vi "InitConfig.vi"() -> ()   [LabVIEW 2014]
uses:
  QMH Fundamentals - Message Cluster.ctl
panel:
  in  "请选择使用的参数":u16(ring) items=["第一条", "第二条", "第三条", "第四条", "第五条"]
  out "保存的参数":string[][](table)
  in  "调用已有参数确定":bool
  in  "调用已有参数返回":bool
  in  "手动确定":bool
  in  "手动示波器试验频率设置(s/条)":dbl=10.0 min=10.0
  in  "示波器试验频率设置(s/条)":dbl=10000.0 min=10000.0
  out "创建的文件路径":string
  in  "请输入需要创建的文件夹名称":string
  in  "路径确定":bool
  in  "自定义试验时间设置(小时)":dbl=0.003 min=0.003
  in  "自定义确定":bool
  in  "自定义返回":bool
  in  "高温老练试验时间设置(小时)":dbl=0.003 min=0.003
  in  "高温老练返回":bool
  in  "高温老练确定":bool
  in  "温循返回":bool
  in  "温循确定":bool
  in  "温循试验时间设置(小时)":dbl=0.003 min=0.003
  in  "单次":bool
  in  "调用已有参数":bool
  in  "手动返回":bool
  in  "返回":bool
  in  "自定义":bool
  in  "高温老练":bool
  in  "温循":bool
  in  "退出":bool
  in  "手动测试":bool
  in  "自动测试":bool
  # "低压元器件应用验证测试系统"
  # "请确定输出文件路径(EXCEL)"
  # "请选择测试类型"
  # "基路径: C:\\output_xls\\"
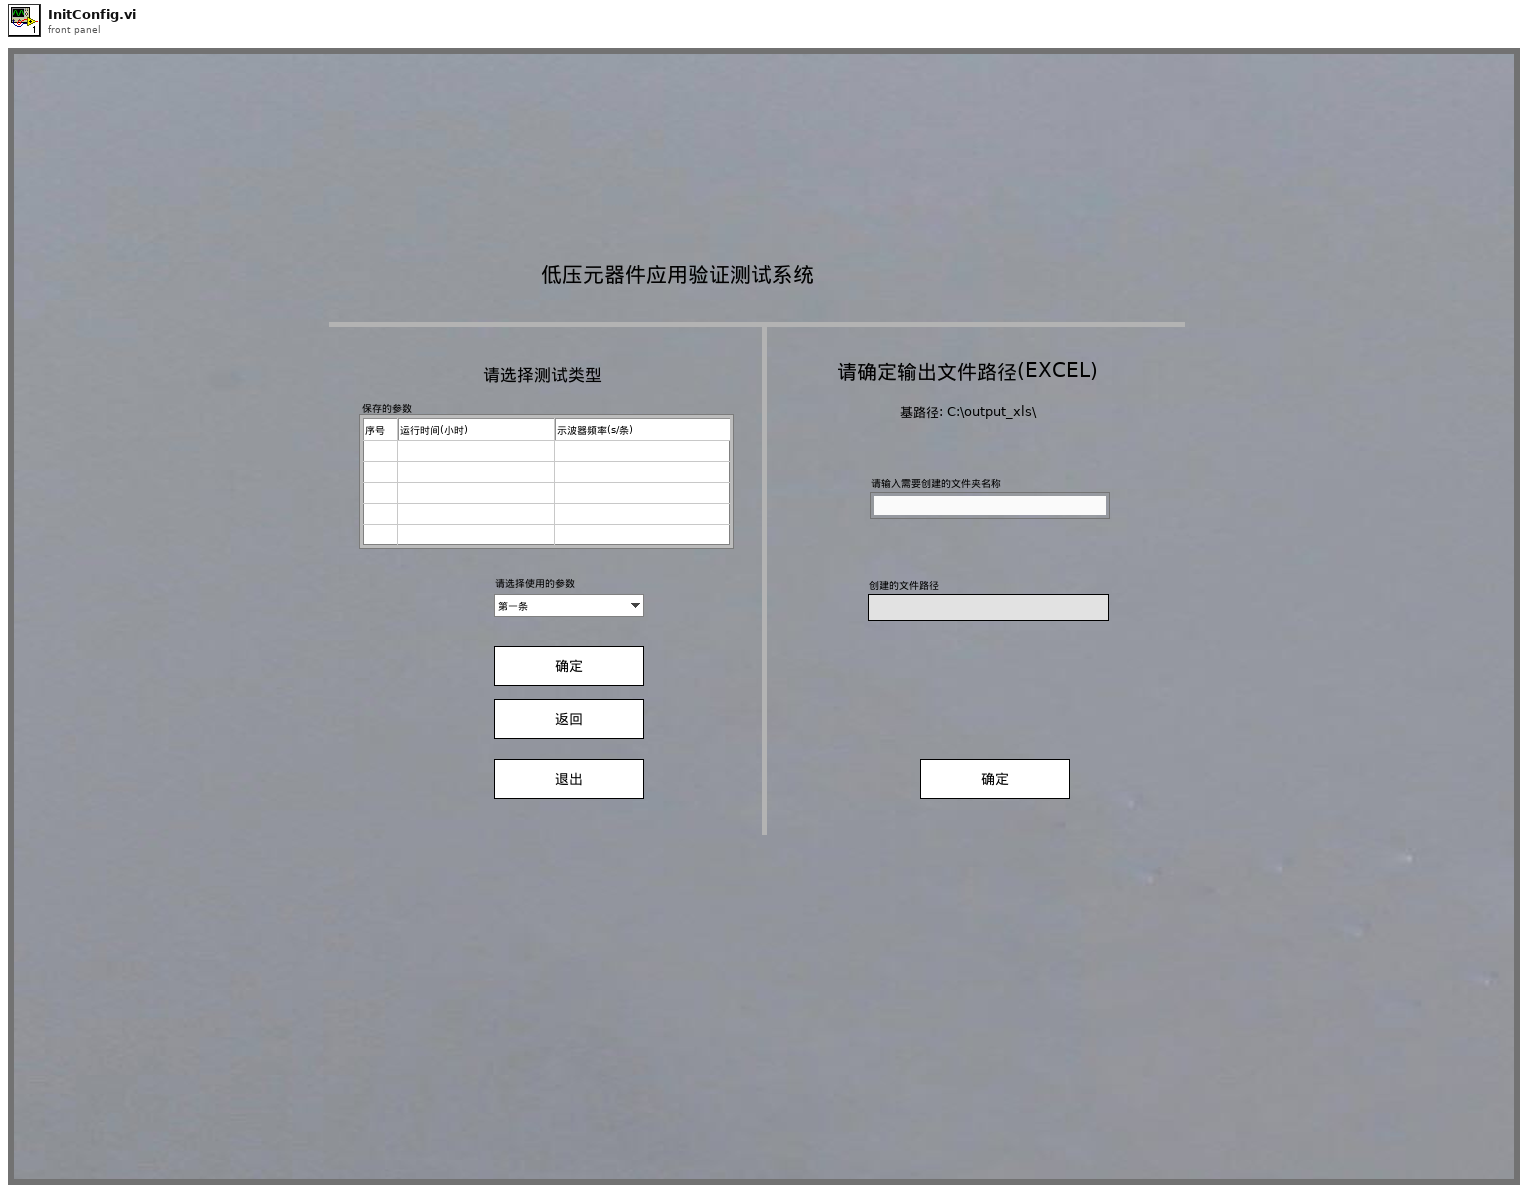
[diagram p1: front panel]
types:
  T1 = typedef "QMH Fundamentals - Message Cluster.ctl" = cluster{"消息":string, "消息数据":variant}
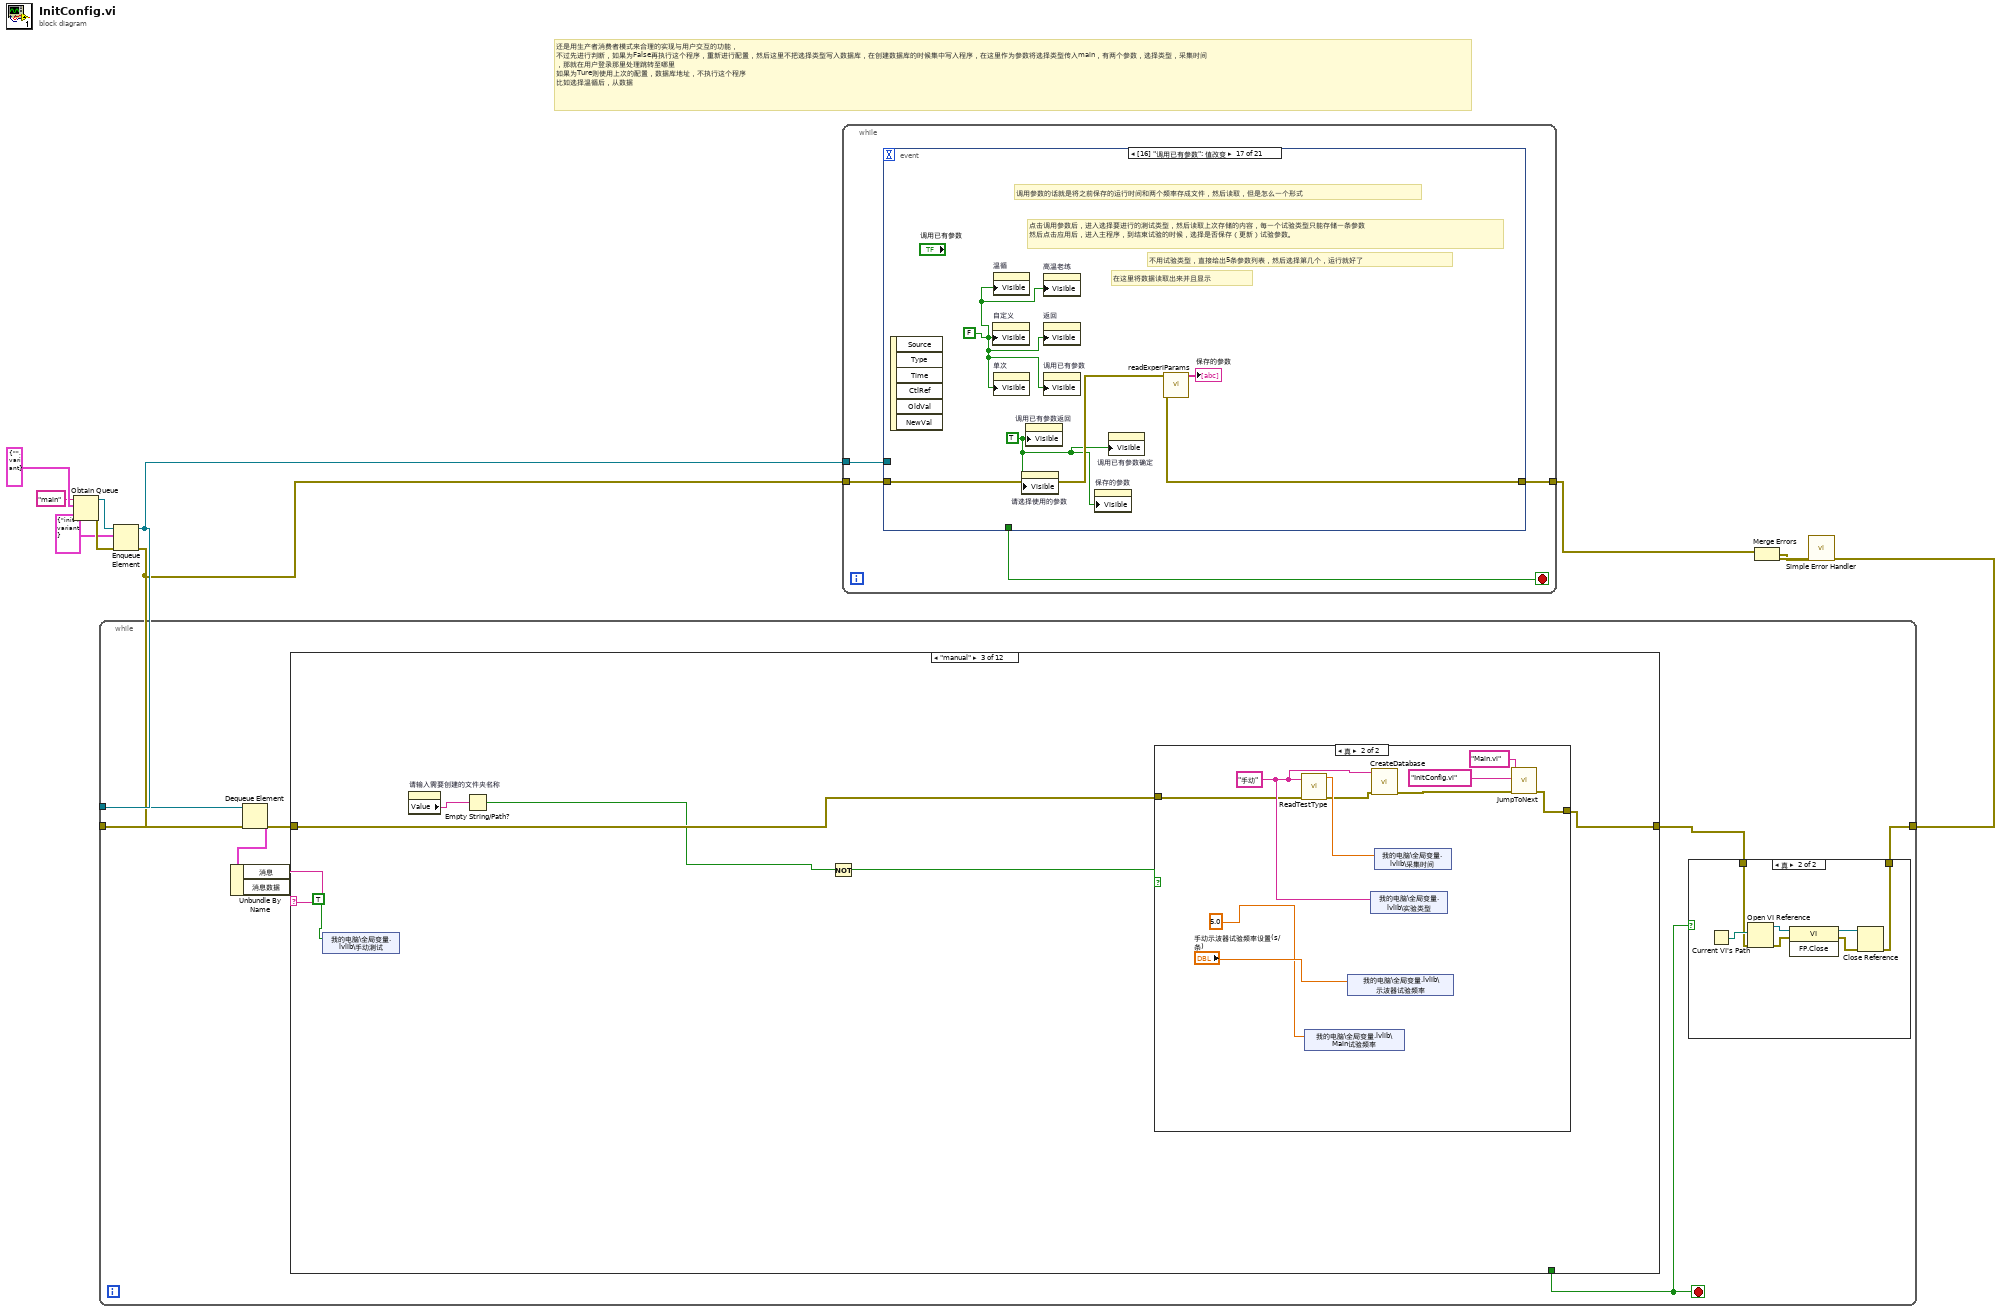
[diagram p0: block diagram]
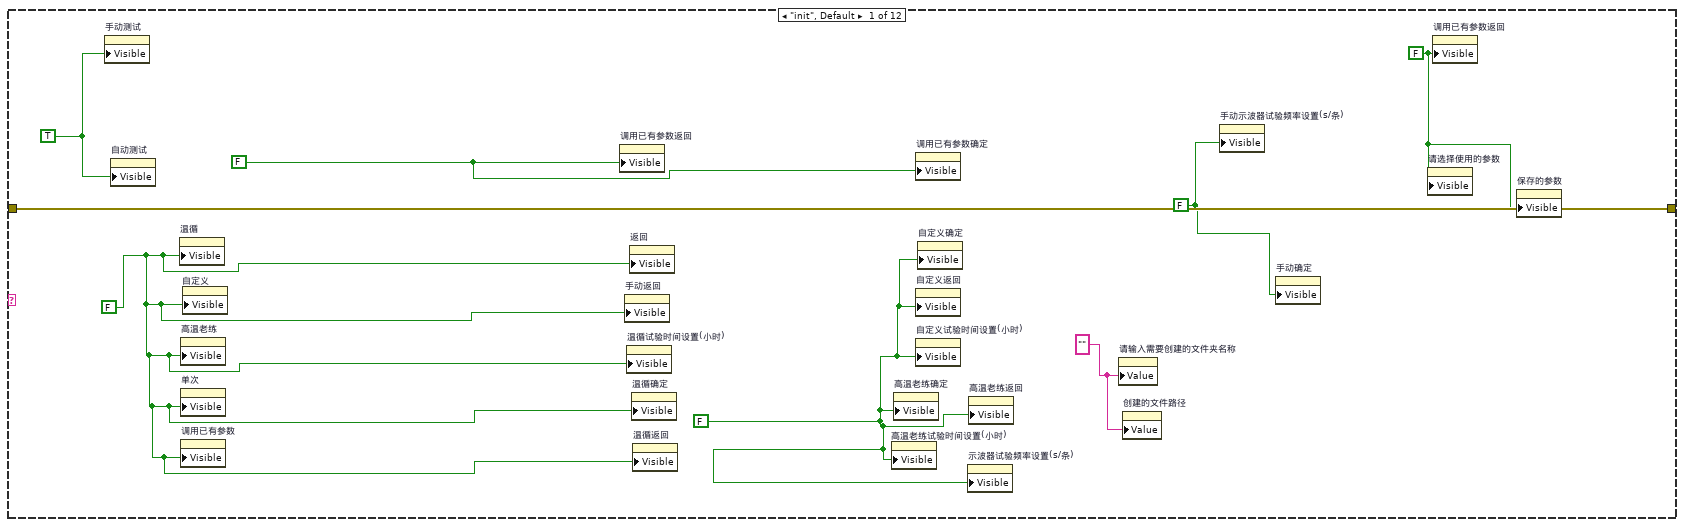
[diagram p3: hidden frame]
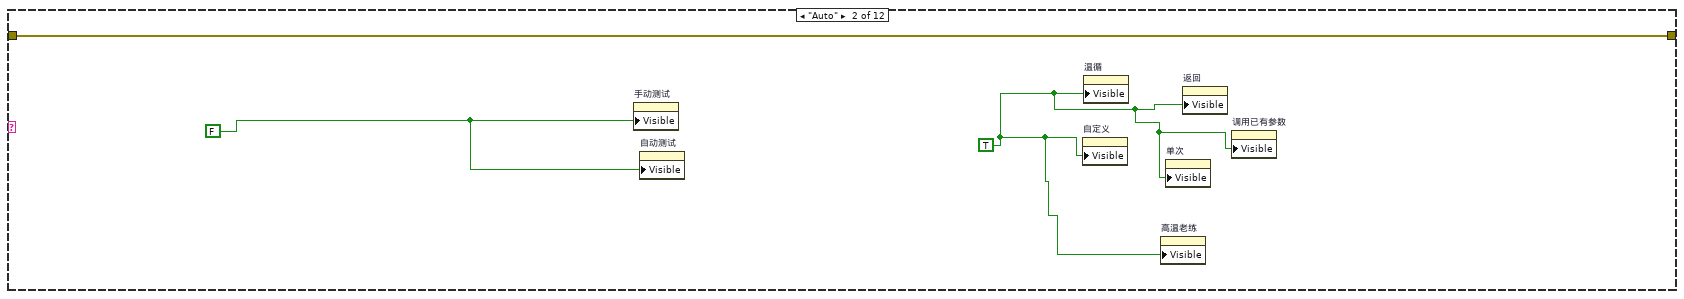
[diagram p4: hidden frame]
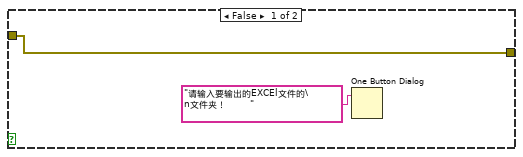
[diagram p5: hidden frame]
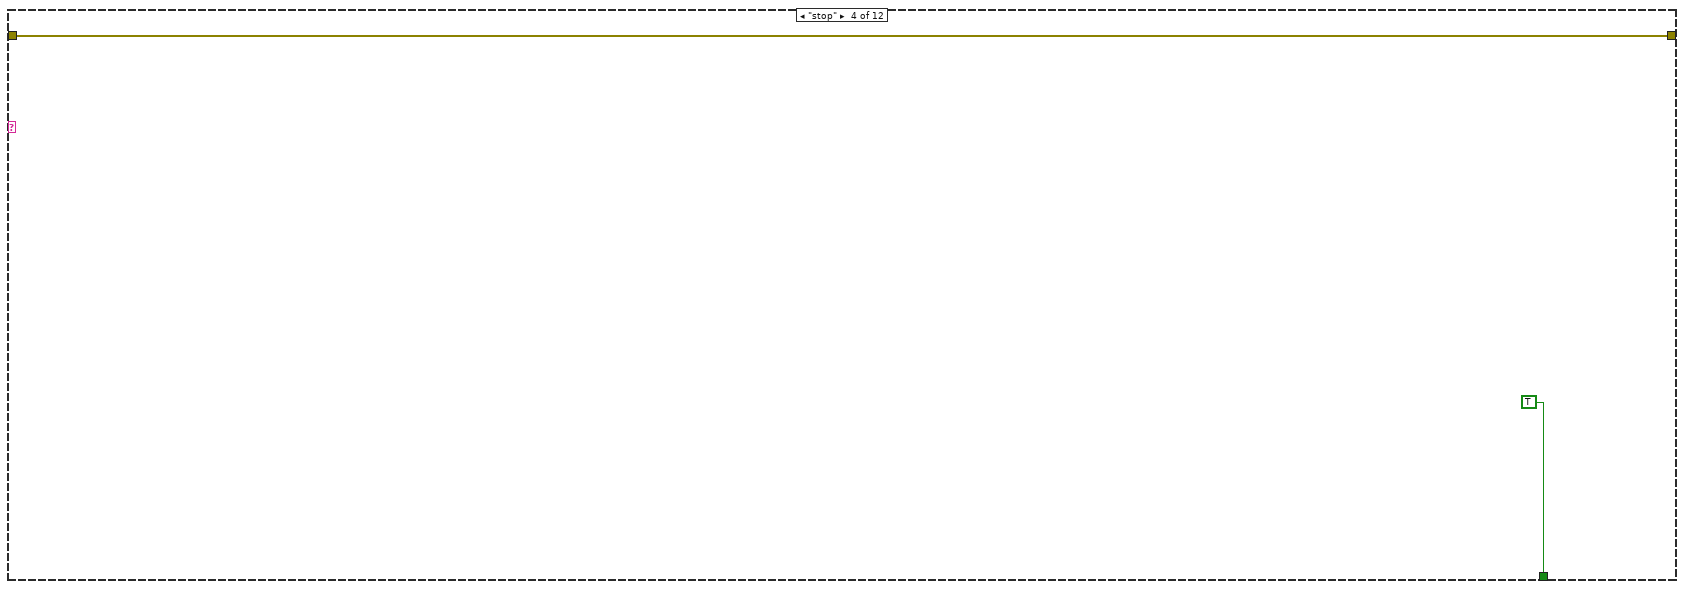
[diagram p6: hidden frame]
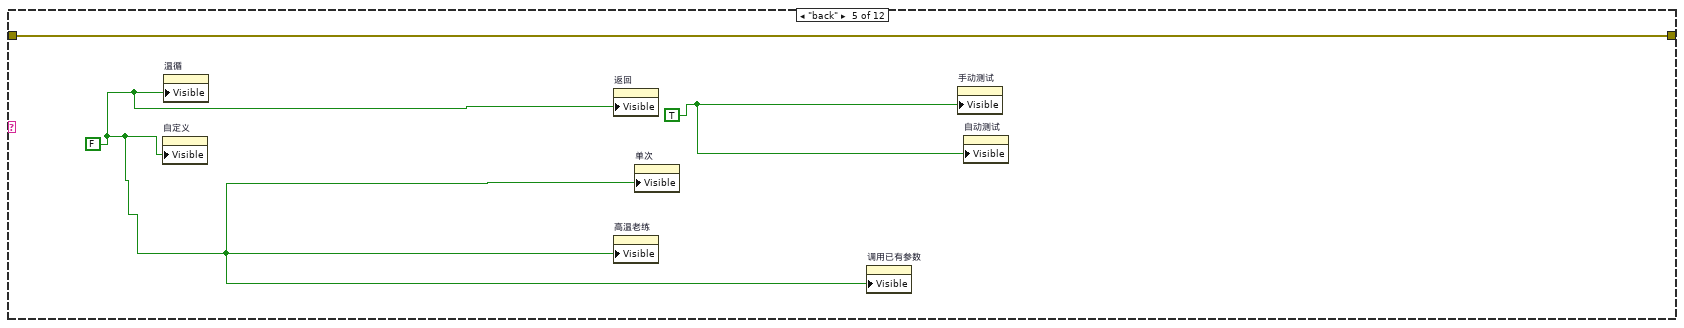
[diagram p7: hidden frame]
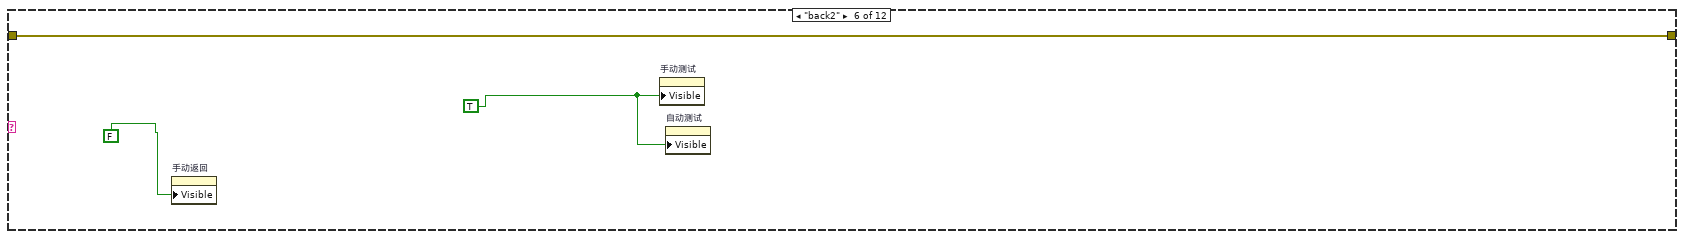
[diagram p8: hidden frame]
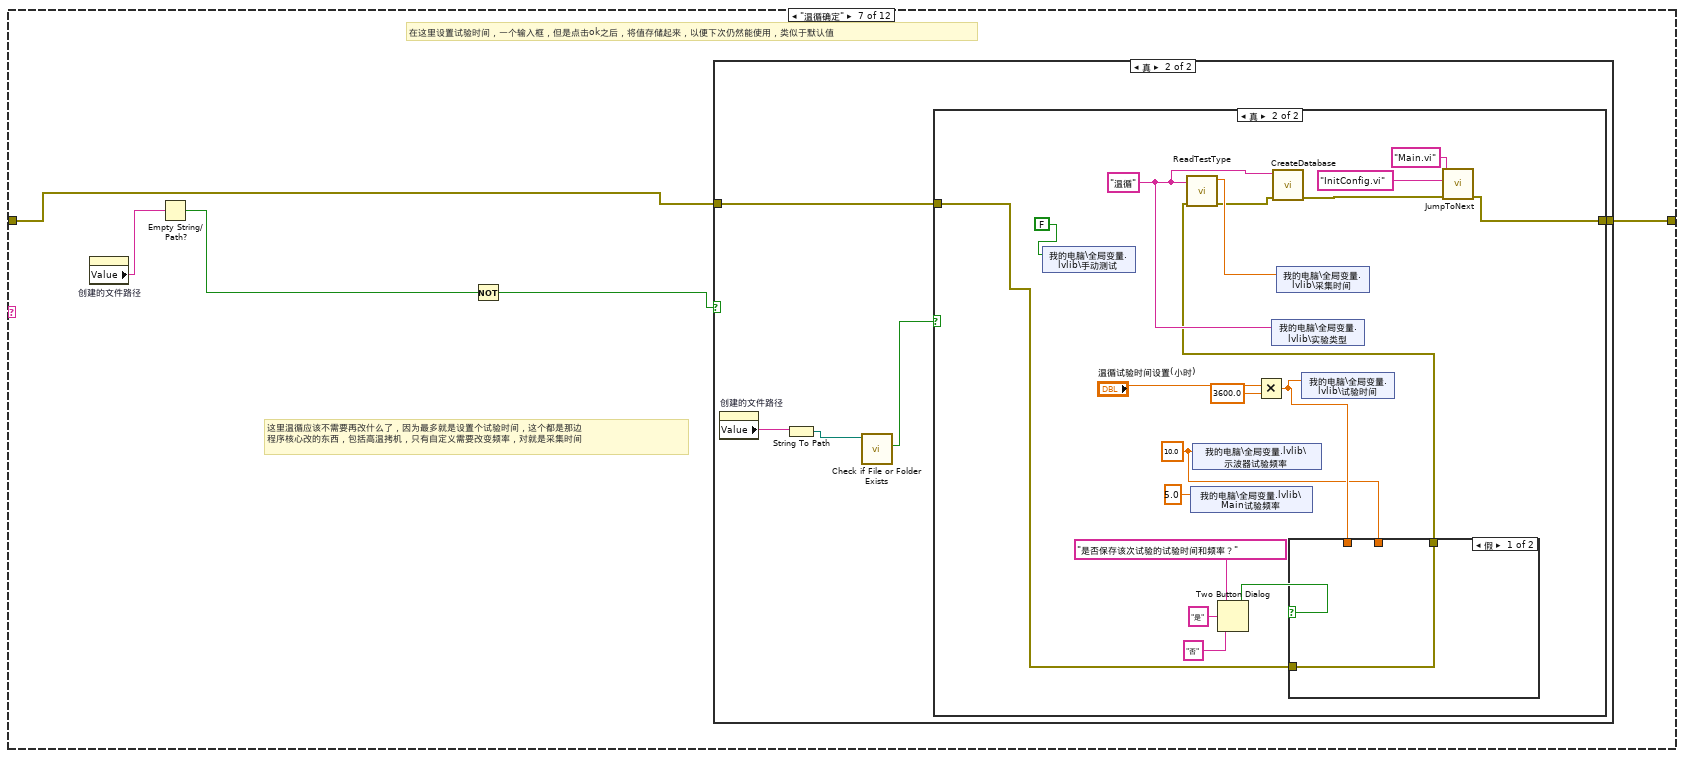
[diagram p9: hidden frame]
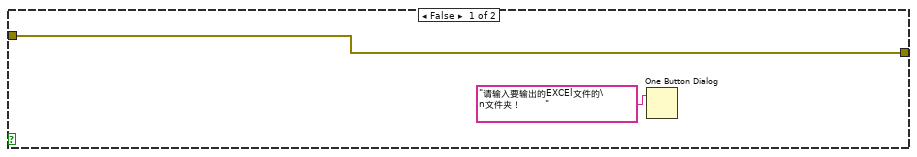
[diagram p10: hidden frame]
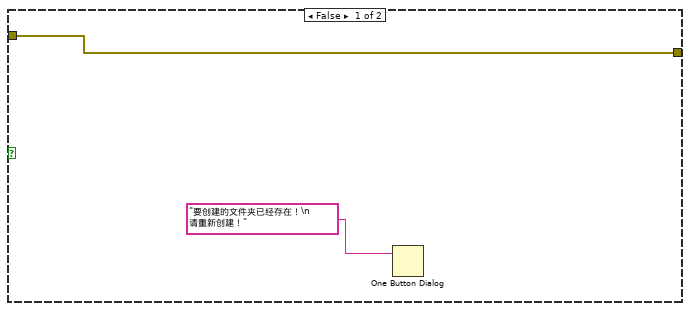
[diagram p11: hidden frame]
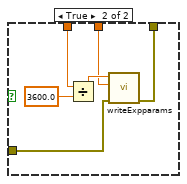
[diagram p12: hidden frame]
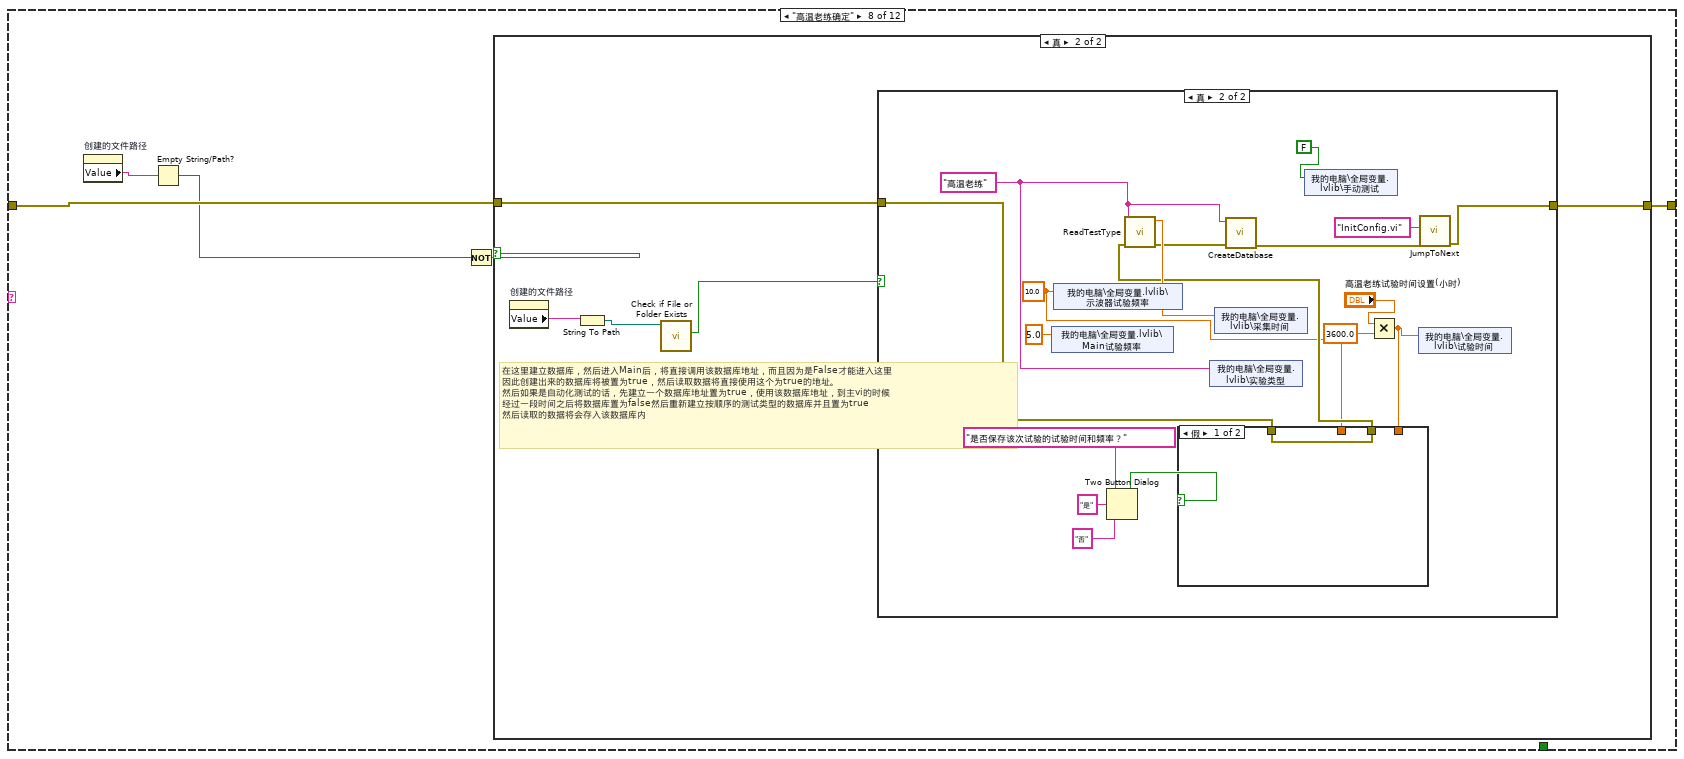
[diagram p13: hidden frame]
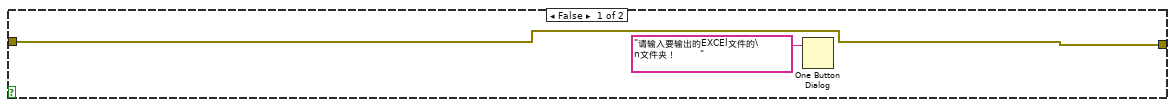
[diagram p14: hidden frame]
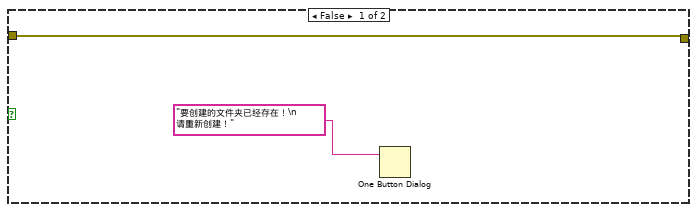
[diagram p15: hidden frame]
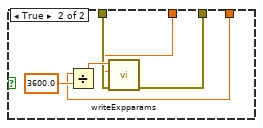
[diagram p16: hidden frame]
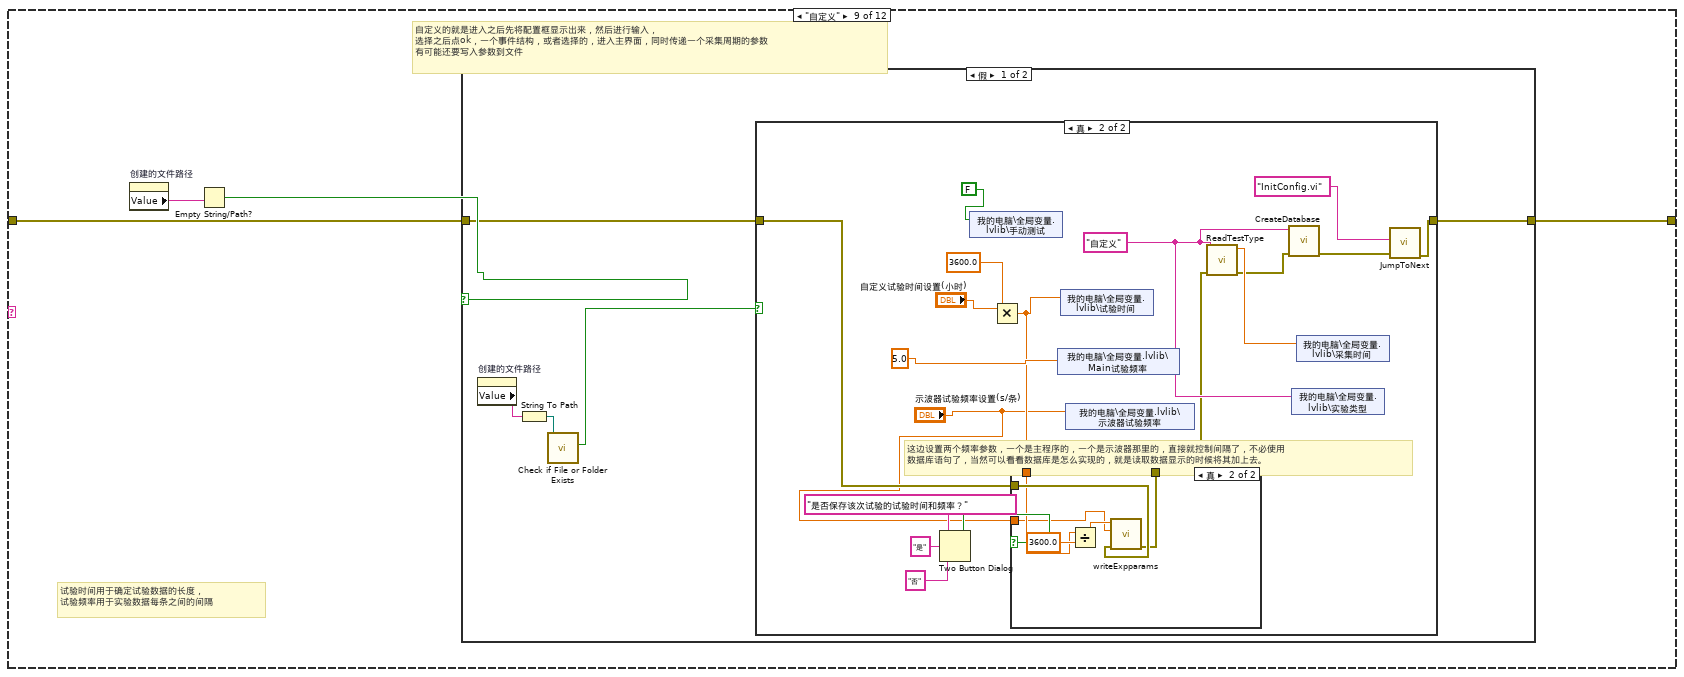
[diagram p17: hidden frame]
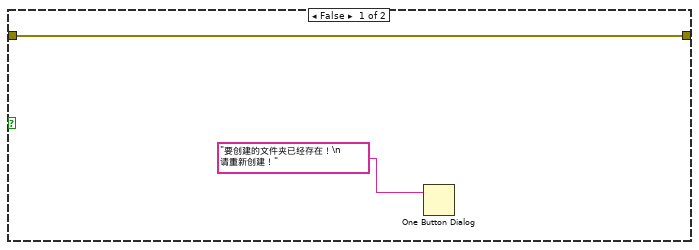
[diagram p18: hidden frame]
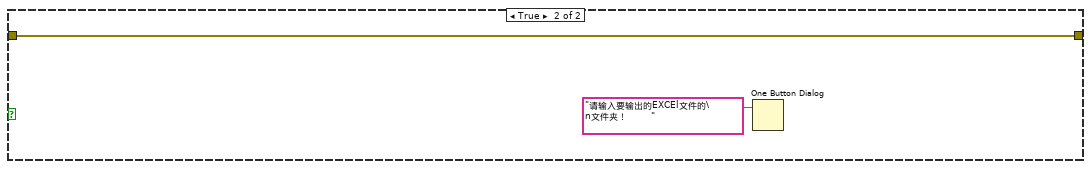
[diagram p20: hidden frame]
diagram:
  # "还是用生产者消费者模式来合理的实现与用户交互的功能，\n不过先进行判断，如果为False再执行这个程序，重新进行配置，然后这里不把选择类型写入数据库，在创建数据库的时候集中写入程序，在这里作为参数将选择类型传入main，有两个参数，选择类型，采集时间\n，那就在用户登录那里处理跳转至哪里\n如果为Ture则使用上次的配置，数据库地址，不执行这个程序\n比如选择温循后，从数据"
  n1 = Obtain Queue(name (unnamed)="main" ("名称（未命名）"), element data type=T1 {"消息"="", "消息数据"=variant} ("消息簇")) -> (queue out=w8:refnum<queue>, error out=w7:errorcluster)  [unwired: 3 in, 1 out]
  n2 = Enqueue Element(queue=w8, element=T1 {"消息"="init", "消息数据"=variant} ("元素"), error in (no error)=w7) -> (queue out=w5:refnum<queue>, error out=w4:errorcluster)  [unwired: 1 in, 1 out]
  n3 = while {
    tunnel: w5 -> [w18]
    tunnel: w4 -> [w17]
    tunnel: [w11] -> w2
    stop <- w13 stop-if-true
    n4 = Dequeue Element(queue=w18, error in (no error)=w17) -> (element=w16:T1, error out=w14:errorcluster)  [unwired: 1 in, 2 out]
    n5 = Unbundle By Name(w16) -> ("消息"=w15:string)  [unwired: 1 out]
    n6 = case shown="\"manual\"" w15 {
      tunnel: w14 -> [w34 w37 w40 w57 w59 w61 w68 w107 w146 w184 w218 w263]
      tunnel: [w34 w37 w39 w57 w59 w61 w67 w106 w145 w183 w219 w268] -> w12
      tunnel: [_ _ _ TRUE _ _ _ _ _ _ _ _] -> w13
      frame "init", Default {
        w28 = FALSE ("可见")
        w27 = FALSE ("可见")
        w29 = FALSE
        w31 = ""
        w30 = FALSE
        w33 = TRUE
        w32 = FALSE
        n7 = property on="手动测试" class="Bool"("Visible"=w33) -> ()  [unwired: 2 in, 2 out]
        n8 = property on="自动测试" class="Bool"("Visible"=w33) -> ()  [unwired: 2 in, 2 out]
        n9 = property on="温循" class="Bool"("Visible"=w32) -> ()  [unwired: 2 in, 2 out]
        n10 = property on="高温老练" class="Bool"("Visible"=w32) -> ()  [unwired: 2 in, 2 out]
        n11 = property on="单次" class="Bool"("Visible"=w32) -> ()  [unwired: 2 in, 2 out]
        n12 = property on="调用已有参数" class="Bool"("Visible"=w32) -> ()  [unwired: 2 in, 2 out]
        n13 = property on="自定义" class="Bool"("Visible"=w32) -> ()  [unwired: 2 in, 2 out]
        n14 = property on="调用已有参数返回" class="Bool"("Visible"=w27) -> ()  [unwired: 2 in, 2 out]
        n15 = property on="手动返回" class="Bool"("Visible"=w32) -> ()  [unwired: 2 in, 2 out]
        n16 = property on="温循试验时间设置(小时)" class="DigNum (严格)"("Visible"=w32) -> ()  [unwired: 2 in, 2 out]
        n17 = property on="返回" class="Bool"("Visible"=w32) -> ()  [unwired: 2 in, 2 out]
        n18 = property on="温循确定" class="Bool"("Visible"=w32) -> ()  [unwired: 2 in, 2 out]
        n19 = property on="温循返回" class="Bool"("Visible"=w32) -> ()  [unwired: 2 in, 2 out]
        n20 = property on="高温老练试验时间设置(小时)" class="DigNum (严格)"("Visible"=w30) -> ()  [unwired: 2 in, 2 out]
        n21 = property on="高温老练确定" class="Bool"("Visible"=w30) -> ()  [unwired: 2 in, 2 out]
        n22 = property on="调用已有参数确定" class="Bool"("Visible"=w27) -> ()  [unwired: 2 in, 2 out]
        n23 = property on="自定义返回" class="Bool"("Visible"=w30) -> ()  [unwired: 2 in, 2 out]
        n24 = property on="自定义试验时间设置(小时)" class="DigNum (严格)"("Visible"=w30) -> ()  [unwired: 2 in, 2 out]
        n25 = property on="自定义确定" class="Bool"("Visible"=w30) -> ()  [unwired: 2 in, 2 out]
        n26 = property on="示波器试验频率设置(s/条)" class="DigNum (严格)"("Visible"=w30) -> ()  [unwired: 2 in, 2 out]
        n27 = property on="高温老练返回" class="Bool"("Visible"=w30) -> ()  [unwired: 2 in, 2 out]
        n28 = property on="请输入需要创建的文件夹名称" class="Str"("Value"=w31) -> ()  [unwired: 2 in, 2 out]
        n29 = property on="创建的文件路径" class="Str"("Value"=w31) -> ()  [unwired: 2 in, 2 out]
        n30 = property on="手动示波器试验频率设置(s/条)" class="DigNum (严格)"("Visible"=w29) -> ()  [unwired: 2 in, 2 out]
        n31 = property on="手动确定" class="Bool"("Visible"=w29) -> ()  [unwired: 2 in, 2 out]
        n32 = property on="请选择使用的参数" class="Ring (严格)"("Visible"=w28) -> ()  [unwired: 2 in, 2 out]
        n33 = property on="调用已有参数返回" class="Bool"("Visible"=w28) -> ()  [unwired: 2 in, 2 out]
        n34 = property on="保存的参数" class="Tbl (严格)"("Visible"=w28) -> ()  [unwired: 2 in, 2 out]
      }
      frame "Auto" {
        w35 = TRUE
        w36 = FALSE
        n35 = property on="手动测试" class="Bool"("Visible"=w36) -> ()  [unwired: 2 in, 2 out]
        n36 = property on="自动测试" class="Bool"("Visible"=w36) -> ()  [unwired: 2 in, 2 out]
        n37 = property on="自定义" class="Bool"("Visible"=w35) -> ()  [unwired: 2 in, 2 out]
        n38 = property on="温循" class="Bool"("Visible"=w35) -> ()  [unwired: 2 in, 2 out]
        n39 = property on="高温老练" class="Bool"("Visible"=w35) -> ()  [unwired: 2 in, 2 out]
        n40 = property on="单次" class="Bool"("Visible"=w35) -> ()  [unwired: 2 in, 2 out]
        n41 = property on="返回" class="Bool"("Visible"=w35) -> ()  [unwired: 2 in, 2 out]
        n42 = property on="调用已有参数" class="Bool"("Visible"=w35) -> ()  [unwired: 2 in, 2 out]
      }
      frame "manual" {
        n43 = shared-variable "我的电脑\\全局变量.lvlib\\手动测试"(TRUE) -> ()  [unwired: 1 in, 1 out]
        n44 = property on="请输入需要创建的文件夹名称" class="Str"() -> ("Value"=w41:string)  [unwired: 2 in, 2 out]
        n45 = Empty String/Path?(string/path=w41) -> (empty?=w38:bool)
        n46 = Not(x=w38) -> (.not. x?=w42:bool)
        n47 = case shown="真" w42 {
          tunnel: [w44 w49] -> w39
          tunnel: w40 -> [w44 w48]
          frame False {
            n48 = One Button Dialog(message="请输入要输出的EXCEl文件的\n文件夹！        " ("消息")) -> ()  [unwired: 1 in, 1 out]
          }
          frame True {
            w52 = "手动"
            n49 = call "ReadTestType.vi"("error in (no error)"=w48, "列名"=w52) -> ("error out"=w53:errorcluster, "输出 1"=w55:dbl)  [unwired: 8 in]
            n50 = shared-variable "我的电脑\\全局变量.lvlib\\Main试验频率"(5.0 ("Main试验频率")) -> ()  [unwired: 1 in, 1 out]
            n51 = shared-variable "我的电脑\\全局变量.lvlib\\示波器试验频率"("手动示波器试验频率设置(s/条)") -> ()  [unwired: 1 in, 1 out]
            n52 = shared-variable "我的电脑\\全局变量.lvlib\\实验类型"(w52) -> ()  [unwired: 1 in, 1 out]
            n53 = call "CreateDatabase.vi"("错误输入（无错误）"=w53, "测试类型"=w52) -> ("error out"=w51:errorcluster)  [unwired: 8 in, 1 out]
            n54 = shared-variable "我的电脑\\全局变量.lvlib\\采集时间"(w55) -> ()  [unwired: 1 in, 1 out]
            n55 = call "JumpToNext.vi"("错误输入（无错误）"=w51, "要关闭的VI"="InitConfig.vi", "要打开的VI"="Main.vi") -> ("错误输出"=w49:errorcluster)  [unwired: 8 in]
          }
        }
      }
      frame "stop" {
      }
      frame "back" {
        w60 = TRUE
        w58 = FALSE
        n56 = property on="自定义" class="Bool"("Visible"=w58) -> ()  [unwired: 2 in, 2 out]
        n57 = property on="温循" class="Bool"("Visible"=w58) -> ()  [unwired: 2 in, 2 out]
        n58 = property on="返回" class="Bool"("Visible"=w58) -> ()  [unwired: 2 in, 2 out]
        n59 = property on="高温老练" class="Bool"("Visible"=w58) -> ()  [unwired: 2 in, 2 out]
        n60 = property on="单次" class="Bool"("Visible"=w58) -> ()  [unwired: 2 in, 2 out]
        n61 = property on="调用已有参数" class="Bool"("Visible"=w58) -> ()  [unwired: 2 in, 2 out]
        n62 = property on="手动测试" class="Bool"("Visible"=w60) -> ()  [unwired: 2 in, 2 out]
        n63 = property on="自动测试" class="Bool"("Visible"=w60) -> ()  [unwired: 2 in, 2 out]
      }
      frame "back2" {
        w62 = TRUE
        n64 = property on="手动返回" class="Bool"("Visible"=FALSE) -> ()  [unwired: 2 in, 2 out]
        n65 = property on="手动测试" class="Bool"("Visible"=w62) -> ()  [unwired: 2 in, 2 out]
        n66 = property on="自动测试" class="Bool"("Visible"=w62) -> ()  [unwired: 2 in, 2 out]
      }
      frame "温循确定" {
        # "这里温循应该不需要再改什么了，因为最多就是设置个试验时间，这个都是那边\n程序核心改的东西，包括高温拷机，只有自定义需要改变频率，对就是采集时间"
        # "在这里设置试验时间，一个输入框，但是点击ok之后，将值存储起来，以便下次仍然能使用，类似于默认值"
        n67 = property on="创建的文件路径" class="Str"() -> ("Value"=w65:string)  [unwired: 2 in, 2 out]
        n68 = Empty String/Path?(string/path=w65) -> (empty?=w66:bool)
        n69 = Not(x=w66) -> (.not. x?=w64:bool)
        n70 = case shown="真" w64 {
          tunnel: w68 -> [w69 w75]
          tunnel: [w69 w74] -> w67
          frame False {
            n71 = One Button Dialog(message="请输入要输出的EXCEl文件的\n文件夹！        " ("消息")) -> ()  [unwired: 1 in, 1 out]
          }
          frame True {
            n72 = property on="创建的文件路径" class="Str"() -> ("Value"=w73:string)  [unwired: 2 in, 2 out]
            n73 = String To Path(string=w73) -> (path=w72:path)
            n74 = call <vilib>:"Check if File or Folder Exists.vi"("path"=w72) -> ("file or folder exists?"=w71:bool)  [unwired: 8 in, 2 out]
            n75 = case shown="真" w71 {
              tunnel: w75 -> [w76 w79]
              tunnel: [w76 w90] -> w74
              frame False {
                n76 = One Button Dialog(message="要创建的文件夹已经存在！\n     请重新创建！") -> ()  [unwired: 1 in, 1 out]
              }
              frame True {
                w80 = 10.0 ("示波器试验频率")
                w93 = "温循"
                n77 = shared-variable "我的电脑\\全局变量.lvlib\\手动测试"(FALSE) -> ()  [unwired: 1 in, 1 out]
                n78 = shared-variable "我的电脑\\全局变量.lvlib\\Main试验频率"(5.0 ("Main试验频率")) -> ()  [unwired: 1 in, 1 out]
                n79 = shared-variable "我的电脑\\全局变量.lvlib\\示波器试验频率"(w80) -> ()  [unwired: 1 in, 1 out]
                n80 = Two Button Dialog(message="是否保存该次试验的试验时间和频率？" ("消息"), 1:"否" ("F按钮名称（“取消”）"), 2:"是" ("T按钮名称（“确定”）")) -> (T button?=w82:bool)
                n81 = Multiply(x="温循试验时间设置(小时)", y=3600.0) -> (x*y=w81:dbl)
                n82 = shared-variable "我的电脑\\全局变量.lvlib\\实验类型"(w93) -> ()  [unwired: 1 in, 1 out]
                n83 = case shown="假" w82 {
                  tunnel: [w97 w101] -> w78
                  tunnel: w81 -> [_ w100]
                  tunnel: w80 -> [_ w99]
                  tunnel: w79 -> [w97 w98]
                  frame False {
                  }
                  frame True {
                    n84 = Divide(x=w100, y=3600.0) -> (x/y=w102:dbl)
                    n85 = call "writeExpparams.vi"("error in (no error)"=w98, "示波器试验频率"=w99, "试验时间"=w102) -> ("error out"=w101:errorcluster)  [unwired: 8 in]
                  }
                }
                n86 = call "ReadTestType.vi"("error in (no error)"=w78, "列名"=w93) -> ("error out"=w94:errorcluster, "输出 1"=w96:dbl)  [unwired: 8 in]
                n87 = call "CreateDatabase.vi"("错误输入（无错误）"=w94, "测试类型"=w93) -> ("error out"=w92:errorcluster)  [unwired: 8 in, 1 out]
                n88 = shared-variable "我的电脑\\全局变量.lvlib\\采集时间"(w96) -> ()  [unwired: 1 in, 1 out]
                n89 = shared-variable "我的电脑\\全局变量.lvlib\\试验时间"(w81) -> ()  [unwired: 1 in, 1 out]
                n90 = call "JumpToNext.vi"("错误输入（无错误）"=w92, "要关闭的VI"="InitConfig.vi", "要打开的VI"="Main.vi") -> ("错误输出"=w90:errorcluster)  [unwired: 8 in]
              }
            }
          }
        }
      }
      frame "高温老练确定" {
        n91 = property on="创建的文件路径" class="Str"() -> ("Value"=w104:string)  [unwired: 2 in, 2 out]
        n92 = Empty String/Path?(string/path=w104) -> (empty?=w105:bool)
        n93 = Not(x=w105) -> (.not. x?=w108:bool)
        n94 = case shown="真" w108 {
          tunnel: w107 -> [w109 w115]
          tunnel: [w109 w114] -> w106
          frame False {
            n95 = One Button Dialog(message="请输入要输出的EXCEl文件的\n文件夹！        " ("消息")) -> ()  [unwired: 1 in, 1 out]
          }
          frame True {
            # "在这里建立数据库，然后进入Main后，将直接调用该数据库地址，而且因为是False才能进入这里\n因此创建出来的数据库将被置为true，然后读取数据将直接使用这个为true的地址。\n然后如果是自动化测试的话，先建立一个数据库地址置为true，使用该数据库地址，到主vi的时候\n经过一段时间之后将数据库置为false然后重新建立按顺序的测试类型的数据库并且置为true\n然后读取的数据将会存入该数据库内"
            n96 = property on="创建的文件路径" class="Str"() -> ("Value"=w113:string)  [unwired: 2 in, 2 out]
            n97 = String To Path(string=w113) -> (path=w112:path)
            n98 = call <vilib>:"Check if File or Folder Exists.vi"("path"=w112) -> ("file or folder exists?"=w111:bool)  [unwired: 8 in, 2 out]
            n99 = case shown="真" w111 {
              tunnel: w115 -> [w116 w121]
              tunnel: [w116 w130] -> w114
              frame False {
                n100 = One Button Dialog(message="要创建的文件夹已经存在！\n     请重新创建！") -> ()  [unwired: 1 in, 1 out]
              }
              frame True {
                w118 = 10.0 ("示波器试验频率")
                w131 = "高温老练"
                n101 = shared-variable "我的电脑\\全局变量.lvlib\\Main试验频率"(5.0 ("Main试验频率")) -> ()  [unwired: 1 in, 1 out]
                n102 = shared-variable "我的电脑\\全局变量.lvlib\\示波器试验频率"(w118) -> ()  [unwired: 1 in, 1 out]
                n103 = Two Button Dialog(message="是否保存该次试验的试验时间和频率？" ("消息"), 1:"否" ("F按钮名称（“取消”）"), 2:"是" ("T按钮名称（“确定”）")) -> (T button?=w122:bool)
                n104 = shared-variable "我的电脑\\全局变量.lvlib\\实验类型"(w131) -> ()  [unwired: 1 in, 1 out]
                n105 = shared-variable "我的电脑\\全局变量.lvlib\\手动测试"(FALSE) -> ()  [unwired: 1 in, 1 out]
                n106 = Multiply(x="高温老练试验时间设置(小时)", y=3600.0) -> (x*y=w119:dbl)
                n107 = case shown="假" w122 {
                  tunnel: [w136 w140] -> w120
                  tunnel: w121 -> [w136 w139]
                  tunnel: w119 -> [_ w138]
                  tunnel: w118 -> [_ w137]
                  frame False {
                  }
                  frame True {
                    n108 = Divide(x=w138, y=3600.0) -> (x/y=w141:dbl)
                    n109 = call "writeExpparams.vi"("error in (no error)"=w139, "示波器试验频率"=w137, "试验时间"=w141) -> ("error out"=w140:errorcluster)  [unwired: 8 in]
                  }
                }
                n110 = call "ReadTestType.vi"("error in (no error)"=w120, "列名"=w131) -> ("error out"=w133:errorcluster, "输出 1"=w135:dbl)  [unwired: 8 in]
                n111 = shared-variable "我的电脑\\全局变量.lvlib\\采集时间"(w135) -> ()  [unwired: 1 in, 1 out]
                n112 = call "CreateDatabase.vi"("错误输入（无错误）"=w133, "测试类型"=w131) -> ("error out"=w132:errorcluster)  [unwired: 8 in, 1 out]
                n113 = shared-variable "我的电脑\\全局变量.lvlib\\试验时间"(w119) -> ()  [unwired: 1 in, 1 out]
                n114 = call "JumpToNext.vi"("错误输入（无错误）"=w132, "要关闭的VI"="InitConfig.vi") -> ("错误输出"=w130:errorcluster)  [unwired: 9 in]
              }
            }
          }
        }
      }
      frame "自定义" {
        # "试验时间用于确定试验数据的长度，\n试验频率用于实验数据每条之间的间隔"
        # "自定义的就是进入之后先将配置框显示出来，然后进行输入，\n选择之后点ok，一个事件结构，或者选择的，进入主界面，同时传递一个采集周期的参数\n有可能还要写入参数到文件"
        n115 = property on="创建的文件路径" class="Str"() -> ("Value"=w143:string)  [unwired: 2 in, 2 out]
        n116 = Empty String/Path?(string/path=w143) -> (empty?=w144:bool)
        n117 = case shown="假" w144 {
          tunnel: w146 -> [w151 w179]
          tunnel: [w150 w179] -> w145
          frame False {
            n118 = property on="创建的文件路径" class="Str"() -> ("Value"=w148:string)  [unwired: 2 in, 2 out]
            n119 = String To Path(string=w148) -> (path=w149:path)
            n120 = call <vilib>:"Check if File or Folder Exists.vi"("path"=w149) -> ("file or folder exists?"=w147:bool)  [unwired: 8 in, 2 out]
            n121 = case shown="真" w147 {
              tunnel: w151 -> [w153 w157]
              tunnel: [w153 w166] -> w150
              frame False {
                n122 = One Button Dialog(message="要创建的文件夹已经存在！\n     请重新创建！") -> ()  [unwired: 1 in, 1 out]
              }
              frame True {
                w167 = "自定义"
                # "这边设置两个频率参数，一个是主程序的，一个是示波器那里的，直接就控制间隔了，不必使用\n数据库语句了，当然可以看看数据库是怎么实现的，就是读取数据显示的时候将其加上去。"
                n123 = Two Button Dialog(message="是否保存该次试验的试验时间和频率？" ("消息"), 1:"否" ("F按钮名称（“取消”）"), 2:"是" ("T按钮名称（“确定”）")) -> (T button?=w158:bool)
                n124 = shared-variable "我的电脑\\全局变量.lvlib\\手动测试"(FALSE) -> ()  [unwired: 1 in, 1 out]
                n125 = Multiply(x="自定义试验时间设置(小时)", y=3600.0) -> (x*y=w155:dbl)
                n126 = case shown="真" w158 {
                  tunnel: w157 -> [w172 w176]
                  tunnel: [w172 w175] -> w156
                  tunnel: w155 -> [_ w174]
                  tunnel: "示波器试验频率设置(s/条)" -> [_ w173]
                  frame False {
                  }
                  frame True {
                    n127 = Divide(x=w174, y=3600.0) -> (x/y=w177:dbl)
                    n128 = call "writeExpparams.vi"("error in (no error)"=w176, "示波器试验频率"=w173, "试验时间"=w177) -> ("error out"=w175:errorcluster)  [unwired: 8 in]
                  }
                }
                n129 = shared-variable "我的电脑\\全局变量.lvlib\\Main试验频率"(5.0 ("Main试验频率")) -> ()  [unwired: 1 in, 1 out]
                n130 = shared-variable "我的电脑\\全局变量.lvlib\\试验时间"(w155) -> ()  [unwired: 1 in, 1 out]
                n131 = shared-variable "我的电脑\\全局变量.lvlib\\示波器试验频率"("示波器试验频率设置(s/条)") -> ()  [unwired: 1 in, 1 out]
                n132 = call "ReadTestType.vi"("error in (no error)"=w156, "列名"=w167) -> ("error out"=w169:errorcluster, "输出 1"=w171:dbl)  [unwired: 8 in]
                n133 = call "CreateDatabase.vi"("错误输入（无错误）"=w169, "测试类型"=w167) -> ("error out"=w168:errorcluster)  [unwired: 8 in, 1 out]
                n134 = shared-variable "我的电脑\\全局变量.lvlib\\实验类型"(w167) -> ()  [unwired: 1 in, 1 out]
                n135 = shared-variable "我的电脑\\全局变量.lvlib\\采集时间"(w171) -> ()  [unwired: 1 in, 1 out]
                n136 = call "JumpToNext.vi"("错误输入（无错误）"=w168, "要关闭的VI"="InitConfig.vi") -> ("错误输出"=w166:errorcluster)  [unwired: 9 in]
              }
            }
          }
          frame True {
            n137 = One Button Dialog(message="请输入要输出的EXCEl文件的\n文件夹！        " ("消息")) -> ()  [unwired: 1 in, 1 out]
          }
        }
      }
      frame "单次" {
        # "试验时间用于确定试验数据的长度，\n试验频率用于实验数据每条之间的间隔"
        # "自定义的就是进入之后先将配置框显示出来，然后进行输入，\n选择之后点ok，一个事件结构，或者选择的，进入主界面，同时传递一个采集周期的参数\n有可能还要写入参数到文件"
        n138 = property on="创建的文件路径" class="Str"() -> ("Value"=w181:string)  [unwired: 2 in, 2 out]
        n139 = Empty String/Path?(string/path=w181) -> (empty?=w182:bool)
        n140 = case shown="假" w182 {
          tunnel: w184 -> [w189 w215]
          tunnel: [w188 w215] -> w183
          frame False {
            # "这边设置两个频率参数，一个是主程序的，一个是示波器那里的，直接就控制间隔了，不必使用\n数据库语句了，当然可以看看数据库是怎么实现的，就是读取数据显示的时候将其加上去。"
            n141 = property on="创建的文件路径" class="Str"() -> ("Value"=w186:string)  [unwired: 2 in, 2 out]
            n142 = String To Path(string=w186) -> (path=w187:path)
            n143 = call <vilib>:"Check if File or Folder Exists.vi"("path"=w187) -> ("file or folder exists?"=w185:bool)  [unwired: 8 in, 2 out]
            n144 = case shown="真" w185 {
              tunnel: w189 -> [w190 w195]
              tunnel: [w190 w202] -> w188
              frame False {
                n145 = One Button Dialog(message="要创建的文件夹已经存在！\n     请重新创建！") -> ()  [unwired: 1 in, 1 out]
              }
              frame True {
                w193 = 170.0 ("试验时间")
                w192 = 10.0 ("示波器试验频率")
                w203 = "单次"
                n146 = shared-variable "我的电脑\\全局变量.lvlib\\手动测试"(FALSE) -> ()  [unwired: 1 in, 1 out]
                n147 = Two Button Dialog(message="是否保存该次试验的试验时间和频率？" ("消息"), 1:"否" ("F按钮名称（“取消”）"), 2:"是" ("T按钮名称（“确定”）")) -> (T button?=w196:bool)
                n148 = shared-variable "我的电脑\\全局变量.lvlib\\Main试验频率"(5.0 ("Main试验频率")) -> ()  [unwired: 1 in, 1 out]
                n149 = shared-variable "我的电脑\\全局变量.lvlib\\试验时间"(w193) -> ()  [unwired: 1 in, 1 out]
                n150 = shared-variable "我的电脑\\全局变量.lvlib\\示波器试验频率"(w192) -> ()  [unwired: 1 in, 1 out]
                n151 = case shown="真" w196 {
                  tunnel: w195 -> [w208 w212]
                  tunnel: [w208 w211] -> w194
                  tunnel: w193 -> [_ w210]
                  tunnel: w192 -> [_ w209]
                  frame False {
                  }
                  frame True {
                    n152 = Divide(x=w210, y=3600.0) -> (x/y=w213:dbl)
                    n153 = call "writeExpparams.vi"("error in (no error)"=w212, "示波器试验频率"=w209, "试验时间"=w213) -> ("error out"=w211:errorcluster)  [unwired: 8 in]
                  }
                }
                n154 = call "ReadTestType.vi"("error in (no error)"=w194, "列名"=w203) -> ("error out"=w205:errorcluster, "输出 1"=w207:dbl)  [unwired: 8 in]
                n155 = call "CreateDatabase.vi"("错误输入（无错误）"=w205, "测试类型"=w203) -> ("error out"=w204:errorcluster)  [unwired: 8 in, 1 out]
                n156 = shared-variable "我的电脑\\全局变量.lvlib\\实验类型"(w203) -> ()  [unwired: 1 in, 1 out]
                n157 = shared-variable "我的电脑\\全局变量.lvlib\\采集时间"(w207) -> ()  [unwired: 1 in, 1 out]
                n158 = call "JumpToNext.vi"("错误输入（无错误）"=w204, "要关闭的VI"="InitConfig.vi") -> ("错误输出"=w202:errorcluster)  [unwired: 9 in]
              }
            }
          }
          frame True {
            n159 = One Button Dialog(message="请输入要输出的EXCEl文件的\n文件夹！        " ("消息")) -> ()  [unwired: 1 in, 1 out]
          }
        }
      }
      frame "调用已有参数" {
        n160 = property on="创建的文件路径" class="Str"() -> ("Value"=w217:string)  [unwired: 2 in, 2 out]
        n161 = Empty String/Path?(string/path=w217) -> (empty?=w220:bool)
        n162 = case shown="假" w220 {
          tunnel: [w225 w251] -> w219
          tunnel: w218 -> [w224 w251]
          frame False {
            n163 = property on="创建的文件路径" class="Str"() -> ("Value"=w223:string)  [unwired: 2 in, 2 out]
            n164 = String To Path(string=w223) -> (path=w222:path)
            n165 = call <vilib>:"Check if File or Folder Exists.vi"("path"=w222) -> ("file or folder exists?"=w221:bool)  [unwired: 8 in, 2 out]
            n166 = case shown="真" w221 {
              tunnel: [w226 w245] -> w225
              tunnel: w224 -> [w226 w243]
              frame False {
                n167 = One Button Dialog(message="要创建的文件夹已经存在！\n     请重新创建！") -> ()  [unwired: 1 in, 1 out]
              }
              frame True {
                w246 = "已有参数"
                # "这边设置两个频率参数，一个是主程序的，一个是示波器那里的，直接就控制间隔了，不必使用\n数据库语句了，当然可以看看数据库是怎么实现的，就是读取数据显示的时候将其加上去。"
                n168 = local read "保存的参数"() -> (w242:string[][])
                n169 = Index Array(array=w242, index (row)="请选择使用的参数") -> (element=w237:string[])  [unwired: 1 in]
                n170 = shared-variable "我的电脑\\全局变量.lvlib\\手动测试"(FALSE) -> ()  [unwired: 1 in, 1 out]
                n171 = Index Array(array=w237, index=3 ("索引")) -> (element=w233:string)
                n172 = Index Array(array=w237, index=2 ("索引")) -> (element=w235:string)
                n173 = Index Array(array=w237, index=1 ("索引")) -> (element=w236:string)
                n174 = Decimal String To Number(string=w233) -> (number=w232:i32)  [unwired: 2 in, 1 out]
                n175 = Decimal String To Number(string=w235) -> (number=w234:i32)  [unwired: 2 in, 1 out]
                n176 = Scan Value(string=w236, format string="%0.5f" ("格式字符串")) -> (value=w231:dbl)  [unwired: 1 in, 1 out]
                n177 = shared-variable "我的电脑\\全局变量.lvlib\\Main试验频率"(w234) -> ()  [unwired: 1 in, 1 out]
                n178 = shared-variable "我的电脑\\全局变量.lvlib\\示波器试验频率"(w232) -> ()  [unwired: 1 in, 1 out]
                n179 = Multiply(x=w231, y=3600) -> (x*y=w229:dbl)
                n180 = shared-variable "我的电脑\\全局变量.lvlib\\试验时间"(w229) -> ()  [unwired: 1 in, 1 out]
                n181 = call "ReadTestType.vi"("error in (no error)"=w243, "列名"=w246) -> ("error out"=w248:errorcluster, "输出 1"=w250:dbl)  [unwired: 8 in]
                n182 = call "CreateDatabase.vi"("错误输入（无错误）"=w248, "测试类型"=w246) -> ("error out"=w247:errorcluster)  [unwired: 8 in, 1 out]
                n183 = shared-variable "我的电脑\\全局变量.lvlib\\实验类型"(w246) -> ()  [unwired: 1 in, 1 out]
                n184 = shared-variable "我的电脑\\全局变量.lvlib\\采集时间"(w250) -> ()  [unwired: 1 in, 1 out]
                n185 = call "JumpToNext.vi"("错误输入（无错误）"=w247, "要关闭的VI"="InitConfig.vi") -> ("错误输出"=w245:errorcluster)  [unwired: 9 in]
              }
            }
          }
          frame True {
            n186 = One Button Dialog(message="请输入要输出的EXCEl文件的\n文件夹！        " ("消息")) -> ()  [unwired: 1 in, 1 out]
          }
        }
      }
      frame "路径确定" {
        w265 = path "C:/output_xls" ("基路径")
        n187 = call <vilib>:"Check if File or Folder Exists.vi"("path"=w265) -> ("file or folder exists?"=w266:bool)  [unwired: 8 in, 2 out]
        n188 = case shown="假" w266 {
          tunnel: w265 -> [w281 w283]
          tunnel: [w280 w283] -> w264
          tunnel: w263 -> [w279 w282]
          tunnel: [w278 w282] -> w260
          frame False {
            n189 = Create Folder(path (use dialog)=w281, error in=w279) -> (created path=w280:path, error out=w278:errorcluster)  [unwired: 1 in, 1 out]
          }
          frame True {
          }
        }
        n190 = Build Path(base path=w264, name or relative path="请输入需要创建的文件夹名称") -> (appended path=w261:path)
        n191 = call <vilib>:"Check if File or Folder Exists.vi"("error in (no error)"=w260, "path"=w261) -> ("error out"=w257:errorcluster, "file or folder exists?"=w259:bool, "dup path"=w258:path)  [unwired: 7 in]
        n192 = Not(x=w259) -> (.not. x?=w254:bool)
        n193 = case shown="真" w254 {
          tunnel: [w271 w276] -> w268
          tunnel: [w272 w275] -> w267
          tunnel: w258 -> [w272 w274]
          tunnel: w257 -> [w271 w273]
          frame False {
            n194 = One Button Dialog(message="文件夹已经存在！\n请重新创建！   " ("消息")) -> ()  [unwired: 1 in, 1 out]
          }
          frame True {
            n195 = Create Folder(prompt (Create Folder)="文件夹创建完毕！" ("提示"), path (use dialog)=w274, error in=w273) -> (created path=w275:path, error out=w276:errorcluster)  [unwired: 1 out]
          }
        }
        n196 = local read "请输入需要创建的文件夹名称"() -> (w262:string)
        n197 = Empty String/Path?(string/path=w262) -> (empty?=w253:bool)
        n198 = Not(x=w253) -> (.not. x?=w256:bool)
        n199 = And(x=w256, y=w254) -> (x .and. y?=w255:bool)
        n200 = case shown="假" w255 {
          tunnel: w267 -> [_ w292]
          tunnel: w253 -> [w284 _]
          frame False {
            n201 = case shown="真" w284 {
              frame False {
              }
              frame True {
                n202 = One Button Dialog(message="未输入Excel存放文件夹！请重新输入！") -> ()  [unwired: 1 in, 1 out]
              }
            }
            n203 = property on="创建的文件路径" class="Str"("Value"="") -> ()  [unwired: 2 in, 2 out]
          }
          frame True {
            n204 = Path To String(path=w292) -> (string=w289:string)
            "创建的文件路径" <- w289
            n205 = Concatenate Strings(w289, "\\") -> (w290:string)
            n206 = shared-variable "我的电脑\\全局变量.lvlib\\输出xls路径"(w290) -> ()  [unwired: 1 in, 1 out]
            n207 = Concatenate Strings("创建Excel存放文件夹成功！" ("消息"), w289) -> (w287:string)
            n208 = One Button Dialog(message=w287) -> ()  [unwired: 1 in, 1 out]
          }
        }
      }
    }
    n209 = case shown="真" w13 {
      tunnel: w12 -> [w19 w21]
      tunnel: [w19 w20] -> w11
      frame False {
      }
      frame True {
        n210 = Current VI's Path() -> (path=w26:path)
        n211 = Open VI Reference(vi path=w26, error in (no error)=w21) -> (vi reference=w25:refnum<vi>, error out=w24:errorcluster)  [unwired: 4 in]
        n212 = invoke class="VI" method="FP.Close"(reference=w25, error in=w24) -> (reference out=w22:refnum<vi>, error out=w23:errorcluster)  [unwired: 1 in, 1 out]
        n213 = Close Reference(reference=w22, error in (no error)=w23) -> (error out=w20:errorcluster)
      }
    }
  }
  n214 = while {
    tunnel: w5 -> [w295]
    tunnel: w4 -> [w294]
    tunnel: [w293] -> w3
    stop <- w296 stop-if-true
    n215 = event shown="[16] \"调用已有参数\": 值改变" {
      selector: _ -> [_ _ _ _ _ _ _ _ _ _ _ _ _ _ _ _ _ _ _ _ _]
      dyn-events: _ -> [_ _ _ _ _ _ _ _ _ _ _ _ _ _ _ _ _ _ _ _ _]
      timeout: _ -> [_ _ _ _ _ _ _ _ _ _ _ _ _ _ _ _ _ _ _ _ _]
      tunnel: [_ _ _ "退出" TRUE _ _ _ _ _ _ _ _ _ _ _ _ _ _ _ _] -> w296
      tunnel: w295 -> [w300 _ w305 w310 w314 w320 _ _ w329 _ _ w339 _ _ w349 _ _ w360 _ w366 w370]
      tunnel: w294 -> [w299 _ w304 w309 w313 w319 _ w325 w328 w331 _ w338 _ _ w348 _ w356 w359 _ w365 w369]
      tunnel: [w297 _ w303 w307 w312 w318 _ w325 w327 w331 _ w337 _ _ w347 _ w355 w358 _ w364 w368] -> w293
      event "自动测试": Value Change {
        n216 = event-data() -> ()  [unwired: 1 in, 6 out]
        n217 = Enqueue Element(queue=w300, element=T1 {"消息"="Auto", "消息数据"=variant} ("元素"), error in (no error)=w299) -> (error out=w297:errorcluster)  [unwired: 1 in, 2 out]
      }
      event "手动测试": Value Change {
        w302 = FALSE
        w301 = TRUE
        n218 = event-data() -> ()  [unwired: 1 in, 6 out]
        n219 = property on="手动返回" class="Bool"("Visible"=w301) -> ()  [unwired: 2 in, 2 out]
        n220 = property on="手动测试" class="Bool"("Visible"=w302) -> ()  [unwired: 2 in, 2 out]
        n221 = property on="手动示波器试验频率设置(s/条)" class="DigNum (严格)"("Visible"=w301) -> ()  [unwired: 2 in, 2 out]
        n222 = property on="自动测试" class="Bool"("Visible"=w302) -> ()  [unwired: 2 in, 2 out]
        n223 = property on="手动确定" class="Bool"("Visible"=w301) -> ()  [unwired: 2 in, 2 out]
      }
      event "手动确定": Value Change {
        n224 = event-data() -> ()  [unwired: 1 in, 6 out]
        n225 = Enqueue Element(queue=w305, element=T1 {"消息"="manual", "消息数据"=variant} ("元素"), error in (no error)=w304) -> (error out=w303:errorcluster)  [unwired: 1 in, 2 out]
      }
      event "退出": Value Change {
        n226 = event-data() -> ()  [unwired: 1 in, 6 out]
        n227 = Enqueue Element At Opposite End(queue=w310, element=T1 {"消息"="stop", "消息数据"=variant} ("元素"), error in (no error)=w309) -> (error out=w307:errorcluster)  [unwired: 1 in, 2 out]
      }
      event Panel Close? {
        n228 = event-data() -> ()  [unwired: 1 in, 4 out]
        n229 = Enqueue Element At Opposite End(queue=w314, element=T1 {"消息"="stop", "消息数据"=variant} ("元素"), error in (no error)=w313) -> (error out=w312:errorcluster)  [unwired: 1 in, 2 out]
        n230 = event-data() -> ()  [unwired: 2 in, 1 out]
      }
      event "返回": Value Change {
        n231 = event-data() -> ()  [unwired: 1 in, 6 out]
        n232 = Enqueue Element(queue=w320, element=T1 {"消息"="back", "消息数据"=variant} ("元素"), error in (no error)=w319) -> (error out=w318:errorcluster)  [unwired: 1 in, 2 out]
      }
      event "手动返回": Value Change {
        w322 = TRUE
        w321 = FALSE
        n233 = event-data() -> ()  [unwired: 1 in, 6 out]
        n234 = property on="手动返回" class="Bool"("Visible"=w321) -> ()  [unwired: 2 in, 2 out]
        n235 = property on="手动测试" class="Bool"("Visible"=w322) -> ()  [unwired: 2 in, 2 out]
        n236 = property on="手动示波器试验频率设置(s/条)" class="DigNum (严格)"("Visible"=w321) -> ()  [unwired: 2 in, 2 out]
        n237 = property on="自动测试" class="Bool"("Visible"=w322) -> ()  [unwired: 2 in, 2 out]
        n238 = property on="手动确定" class="Bool"("Visible"=w321) -> ()  [unwired: 2 in, 2 out]
      }
      event "温循": Value Change {
        w324 = TRUE
        w326 = FALSE
        # "先将其他按钮进行隐藏，然后点击温循确定的时候再跳转"
        n239 = event-data() -> ()  [unwired: 1 in, 6 out]
        n240 = property on="自定义" class="Bool"("Visible"=w326) -> ()  [unwired: 2 in, 2 out]
        n241 = property on="温循" class="Bool"("Visible"=w326) -> ()  [unwired: 2 in, 2 out]
        n242 = property on="单次" class="Bool"("Visible"=w326) -> ()  [unwired: 2 in, 2 out]
        n243 = property on="温循试验时间设置(小时)" class="DigNum (严格)"("Visible"=w324) -> ()  [unwired: 2 in, 2 out]
        n244 = property on="温循确定" class="Bool"("Visible"=w324) -> ()  [unwired: 2 in, 2 out]
        n245 = property on="高温老练" class="Bool"("Visible"=w326) -> ()  [unwired: 2 in, 2 out]
        n246 = property on="返回" class="Bool"("Visible"=w326) -> ()  [unwired: 2 in, 2 out]
        n247 = property on="调用已有参数" class="Bool"("Visible"=w326) -> ()  [unwired: 2 in, 2 out]
        n248 = property on="温循返回" class="Bool"("Visible"=w324) -> ()  [unwired: 2 in, 2 out]
        n249 = property on="温循试验时间设置(小时)" class="DigNum (严格)"("Value"=500.0 ("温循试验时间设置(s)")) -> ()  [unwired: 2 in, 2 out]
      }
      event "温循确定": Value Change {
        n250 = event-data() -> ()  [unwired: 1 in, 6 out]
        n251 = Enqueue Element(queue=w329, element=T1 {"消息"="温循确定", "消息数据"=variant} ("元素"), error in (no error)=w328) -> (error out=w327:errorcluster)  [unwired: 1 in, 2 out]
      }
      event "温循返回": Value Change {
        w332 = FALSE
        w333 = TRUE
        n252 = event-data() -> ()  [unwired: 1 in, 6 out]
        n253 = property on="自定义" class="Bool"("Visible"=w333) -> ()  [unwired: 2 in, 2 out]
        n254 = property on="温循" class="Bool"("Visible"=w333) -> ()  [unwired: 2 in, 2 out]
        n255 = property on="单次" class="Bool"("Visible"=w333) -> ()  [unwired: 2 in, 2 out]
        n256 = property on="温循试验时间设置(小时)" class="DigNum (严格)"("Visible"=w332) -> ()  [unwired: 2 in, 2 out]
        n257 = property on="温循确定" class="Bool"("Visible"=w332) -> ()  [unwired: 2 in, 2 out]
        n258 = property on="高温老练" class="Bool"("Visible"=w333) -> ()  [unwired: 2 in, 2 out]
        n259 = property on="返回" class="Bool"("Visible"=w333) -> ()  [unwired: 2 in, 2 out]
        n260 = property on="调用已有参数" class="Bool"("Visible"=w333) -> ()  [unwired: 2 in, 2 out]
        n261 = property on="温循返回" class="Bool"("Visible"=w332) -> ()  [unwired: 2 in, 2 out]
      }
      event "高温老练": Value Change {
        w336 = TRUE
        w335 = FALSE
        n262 = event-data() -> ()  [unwired: 1 in, 6 out]
        n263 = property on="高温老练试验时间设置(小时)" class="DigNum (严格)"("Visible"=w336) -> ()  [unwired: 2 in, 2 out]
        n264 = property on="自定义" class="Bool"("Visible"=w335) -> ()  [unwired: 2 in, 2 out]
        n265 = property on="高温老练确定" class="Bool"("Visible"=w336) -> ()  [unwired: 2 in, 2 out]
        n266 = property on="温循" class="Bool"("Visible"=w335) -> ()  [unwired: 2 in, 2 out]
        n267 = property on="单次" class="Bool"("Visible"=w335) -> ()  [unwired: 2 in, 2 out]
        n268 = property on="高温老练" class="Bool"("Visible"=w335) -> ()  [unwired: 2 in, 2 out]
        n269 = property on="返回" class="Bool"("Visible"=w335) -> ()  [unwired: 2 in, 2 out]
        n270 = property on="调用已有参数" class="Bool"("Visible"=w335) -> ()  [unwired: 2 in, 2 out]
        n271 = property on="高温老练返回" class="Bool"("Visible"=w336) -> ()  [unwired: 2 in, 2 out]
        n272 = property on="高温老练试验时间设置(小时)" class="DigNum (严格)"("Value"=1000.0 ("高温老练试验时间设置(s)")) -> ()  [unwired: 2 in, 2 out]
      }
      event "高温老练确定": Value Change {
        n273 = event-data() -> ()  [unwired: 1 in, 6 out]
        n274 = Enqueue Element(queue=w339, element=T1 {"消息"="高温老练确定", "消息数据"=variant} ("元素"), error in (no error)=w338) -> (error out=w337:errorcluster)  [unwired: 1 in, 2 out]
      }
      event "高温老练返回": Value Change {
        w342 = FALSE
        w341 = TRUE
        n275 = event-data() -> ()  [unwired: 1 in, 6 out]
        n276 = property on="高温老练试验时间设置(小时)" class="DigNum (严格)"("Visible"=w342) -> ()  [unwired: 2 in, 2 out]
        n277 = property on="自定义" class="Bool"("Visible"=w341) -> ()  [unwired: 2 in, 2 out]
        n278 = property on="高温老练确定" class="Bool"("Visible"=w342) -> ()  [unwired: 2 in, 2 out]
        n279 = property on="温循" class="Bool"("Visible"=w341) -> ()  [unwired: 2 in, 2 out]
        n280 = property on="单次" class="Bool"("Visible"=w341) -> ()  [unwired: 2 in, 2 out]
        n281 = property on="高温老练" class="Bool"("Visible"=w341) -> ()  [unwired: 2 in, 2 out]
        n282 = property on="返回" class="Bool"("Visible"=w341) -> ()  [unwired: 2 in, 2 out]
        n283 = property on="调用已有参数" class="Bool"("Visible"=w341) -> ()  [unwired: 2 in, 2 out]
        n284 = property on="高温老练返回" class="Bool"("Visible"=w342) -> ()  [unwired: 2 in, 2 out]
      }
      event "自定义": Value Change {
        (unwired) 5.0 ("自定义试验频率设置(s/条)")
        w343 = TRUE
        w346 = FALSE
        n285 = event-data() -> ()  [unwired: 1 in, 6 out]
        n286 = property on="自定义" class="Bool"("Visible"=w346) -> ()  [unwired: 2 in, 2 out]
        n287 = property on="温循" class="Bool"("Visible"=w346) -> ()  [unwired: 2 in, 2 out]
        n288 = property on="单次" class="Bool"("Visible"=w346) -> ()  [unwired: 2 in, 2 out]
        n289 = property on="高温老练" class="Bool"("Visible"=w346) -> ()  [unwired: 2 in, 2 out]
        n290 = property on="返回" class="Bool"("Visible"=w346) -> ()  [unwired: 2 in, 2 out]
        n291 = property on="调用已有参数" class="Bool"("Visible"=w346) -> ()  [unwired: 2 in, 2 out]
        n292 = property on="自定义返回" class="Bool"("Visible"=w343) -> ()  [unwired: 2 in, 2 out]
        n293 = property on="自定义试验时间设置(小时)" class="DigNum (严格)"("Visible"=w343) -> ()  [unwired: 2 in, 2 out]
        n294 = property on="自定义确定" class="Bool"("Visible"=w343) -> ()  [unwired: 2 in, 2 out]
        n295 = property on="示波器试验频率设置(s/条)" class="DigNum (严格)"("Visible"=w343) -> ()  [unwired: 2 in, 2 out]
        n296 = property on="示波器试验频率设置(s/条)" class="DigNum (严格)"("Value"=10.0) -> ()  [unwired: 2 in, 2 out]
        n297 = property on="自定义试验时间设置(小时)" class="DigNum (严格)"("Value"=500.0 ("自定义试验时间设置(s)")) -> ()  [unwired: 2 in, 2 out]
      }
      event "自定义确定": Value Change {
        n298 = event-data() -> ()  [unwired: 1 in, 6 out]
        n299 = Enqueue Element(queue=w349, element=T1 {"消息"="自定义", "消息数据"=variant} ("元素"), error in (no error)=w348) -> (error out=w347:errorcluster)  [unwired: 1 in, 2 out]
      }
      event "自定义返回": Value Change {
        w351 = FALSE
        w352 = TRUE
        n300 = event-data() -> ()  [unwired: 1 in, 6 out]
        n301 = property on="自定义" class="Bool"("Visible"=w352) -> ()  [unwired: 2 in, 2 out]
        n302 = property on="温循" class="Bool"("Visible"=w352) -> ()  [unwired: 2 in, 2 out]
        n303 = property on="单次" class="Bool"("Visible"=w352) -> ()  [unwired: 2 in, 2 out]
        n304 = property on="高温老练" class="Bool"("Visible"=w352) -> ()  [unwired: 2 in, 2 out]
        n305 = property on="返回" class="Bool"("Visible"=w352) -> ()  [unwired: 2 in, 2 out]
        n306 = property on="调用已有参数" class="Bool"("Visible"=w352) -> ()  [unwired: 2 in, 2 out]
        n307 = property on="自定义返回" class="Bool"("Visible"=w351) -> ()  [unwired: 2 in, 2 out]
        n308 = property on="自定义试验时间设置(小时)" class="DigNum (严格)"("Visible"=w351) -> ()  [unwired: 2 in, 2 out]
        n309 = property on="示波器试验频率设置(s/条)" class="DigNum (严格)"("Visible"=w351) -> ()  [unwired: 2 in, 2 out]
        n310 = property on="自定义确定" class="Bool"("Visible"=w351) -> ()  [unwired: 2 in, 2 out]
      }
      event "调用已有参数": Value Change {
        w353 = TRUE ("可见")
        w357 = FALSE
        # "在这里将数据读取出来并且显示"
        # "不用试验类型，直接给出5条参数列表，然后选择第几个，运行就好了"
        # "点击调用参数后，进入选择要进行的测试类型，然后读取上次存储的内容，每一个试验类型只能存储一条参数\n然后点击应用后，进入主程序，到结束试验的时候，选择是否保存（更新）试验参数。"
        # "调用参数的话就是将之前保存的运行时间和两个频率存成文件，然后读取，但是怎么一个形式"
        n311 = event-data() -> ()  [unwired: 1 in, 6 out]
        n312 = property on="自定义" class="Bool"("Visible"=w357) -> ()  [unwired: 2 in, 2 out]
        n313 = property on="温循" class="Bool"("Visible"=w357) -> ()  [unwired: 2 in, 2 out]
        n314 = property on="单次" class="Bool"("Visible"=w357) -> ()  [unwired: 2 in, 2 out]
        n315 = property on="请选择使用的参数" class="Ring (严格)"("Visible"=w353) -> ()  [unwired: 2 in, 2 out]
        n316 = property on="调用已有参数返回" class="Bool"("Visible"=w353) -> ()  [unwired: 2 in, 2 out]
        n317 = property on="高温老练" class="Bool"("Visible"=w357) -> ()  [unwired: 2 in, 2 out]
        n318 = property on="返回" class="Bool"("Visible"=w357) -> ()  [unwired: 2 in, 2 out]
        n319 = property on="调用已有参数" class="Bool"("Visible"=w357) -> ()  [unwired: 2 in, 2 out]
        n320 = property on="保存的参数" class="Tbl (严格)"("Visible"=w353) -> ()  [unwired: 2 in, 2 out]
        n321 = property on="调用已有参数确定" class="Bool"("Visible"=w353) -> ()  [unwired: 2 in, 2 out]
        n322 = call "readExperiParams.vi"("error in (no error)"=w356) -> ("表格控件"=→"保存的参数":string[][], "error out"=w355:errorcluster)  [unwired: 9 in]
      }
      event "调用已有参数确定": Value Change {
        n323 = event-data() -> ()  [unwired: 1 in, 6 out]
        n324 = Enqueue Element(queue=w360, element=T1 {"消息"="调用已有参数", "消息数据"=variant} ("元素"), error in (no error)=w359) -> (error out=w358:errorcluster)  [unwired: 1 in, 2 out]
      }
      event "调用已有参数返回": Value Change {
        w362 = FALSE ("可见")
        w363 = TRUE
        n325 = event-data() -> ()  [unwired: 1 in, 6 out]
        n326 = property on="自定义" class="Bool"("Visible"=w363) -> ()  [unwired: 2 in, 2 out]
        n327 = property on="温循" class="Bool"("Visible"=w363) -> ()  [unwired: 2 in, 2 out]
        n328 = property on="单次" class="Bool"("Visible"=w363) -> ()  [unwired: 2 in, 2 out]
        n329 = property on="高温老练" class="Bool"("Visible"=w363) -> ()  [unwired: 2 in, 2 out]
        n330 = property on="返回" class="Bool"("Visible"=w363) -> ()  [unwired: 2 in, 2 out]
        n331 = property on="调用已有参数" class="Bool"("Visible"=w363) -> ()  [unwired: 2 in, 2 out]
        n332 = property on="请选择使用的参数" class="Ring (严格)"("Visible"=w362) -> ()  [unwired: 2 in, 2 out]
        n333 = property on="调用已有参数返回" class="Bool"("Visible"=w362) -> ()  [unwired: 2 in, 2 out]
        n334 = property on="调用已有参数确定" class="Bool"("Visible"=w362) -> ()  [unwired: 2 in, 2 out]
        n335 = property on="保存的参数" class="Tbl (严格)"("Visible"=w362) -> ()  [unwired: 2 in, 2 out]
      }
      event "单次": Value Change {
        n336 = event-data() -> ()  [unwired: 1 in, 6 out]
        n337 = Enqueue Element(queue=w366, element=T1 {"消息"="单次", "消息数据"=variant} ("元素"), error in (no error)=w365) -> (error out=w364:errorcluster)  [unwired: 1 in, 2 out]
      }
      event "路径确定": Value Change {
        n338 = event-data() -> ()  [unwired: 1 in, 6 out]
        n339 = Enqueue Element(queue=w370, element=T1 {"消息"="路径确定", "消息数据"=variant} ("元素"), error in (no error)=w369) -> (error out=w368:errorcluster)  [unwired: 1 in, 2 out]
      }
    }
  }
  n340 = Merge Errors(w3, w2) -> (w1:errorcluster)
  n341 = call <vilib>:"Simple Error Handler.vi"("error in (no error)"=w1) -> ()  [unwired: 4 in, 5 out]
